vi "Motion Profile Paths.vi"   [LabVIEW 2019]
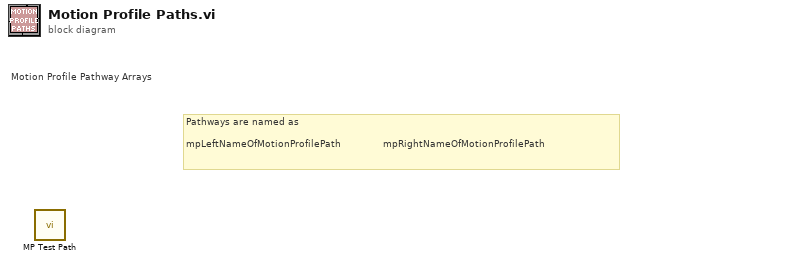
[diagram p0: block diagram]
diagram:
  # "Pathways are named as\n\nmpLeftNameOfMotionProfilePath              mpRightNameOfMotionProfilePath"
  # "Motion Profile Pathway Arrays"
  n1 = call "MP Test Path.vi"() -> ()  [unwired: 12 in]
